vi "MaxValue.vi"(10 "NewValue":fxp<+/-,24,1>, 11 "DataValid":bool) -> (3 "Max":fxp<+/-,24,1>)   [LabVIEW 2018]
uses:
  <instrlib>/_niInstr/Basic Elements/v1/FPGA/Private/Count Up U8.vi
  <instrlib>/_niInstr/Basic Elements/v1/FPGA/niInstr Basic Elements v1 FPGA.lvlib
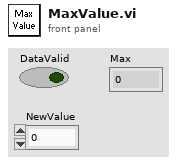
[diagram p1: front panel]
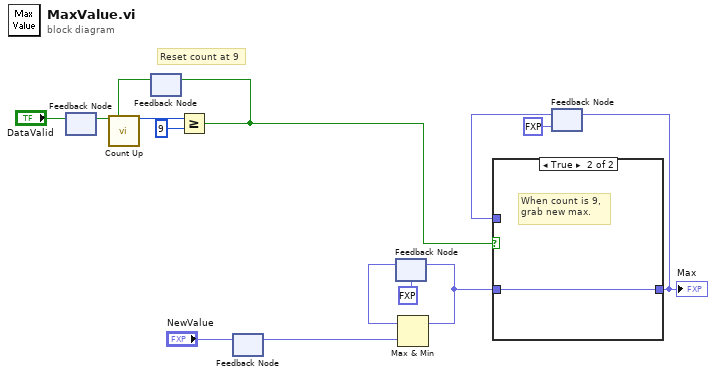
[diagram p0: block diagram]
diagram:
  # "Reset count at 9"
  n1 = feedback-in #1("DataValid") -> ()
  n2 = feedback #1() -> (w7:bool)  [unwired: 1 in]
  n3 = feedback #2() -> (w8:bool)  [unwired: 1 in]
  n4 = call-poly <instrlib>:"Count Up.vi"("increment"=w7, "reset"=w8) -> ("count out"=w10:u8)  [unwired: 13 in]
  n5 = Greater Or Equal?(x=w10, y=u8 9) -> (x >= y?=w4:bool)
  n6 = feedback-in #2(w4) -> ()
  n7 = feedback-in #3("NewValue") -> ()
  n8 = feedback #3() -> (w6:fxp<+/-,24,1>)  [unwired: 1 in]
  n9 = feedback #4(fxp<+/-,24,1> 0.0) -> (w13:fxp<+/-,24,1>)
  n10 = Max & Min(x=w13, y=w6) -> (max(x,y)=w5:fxp<+/-,24,1>)  [unwired: 1 out]
  n11 = feedback-in #4(w5) -> ()
  n12 = feedback #5(fxp<+/-,24,1> 0.0) -> (w2:fxp<+/-,24,1>)
  n13 = case shown="True" w4 {
    tunnel: w5 -> [_ w16]
    tunnel: [w15 w16] -> w3
    tunnel: w2 -> [w15 _]
    frame False {
      # "When less than 9,\nrepeat previous max."
    }
    frame True {
      # "When count is 9,\ngrab new max."
    }
  }
  "Max" <- w3
  n14 = feedback-in #5(w3) -> ()
